vi "Example.vi"() -> ()   [LabVIEW 2016, in "SLSC Switch.lvlib"]
uses:
  SLSC Switch.lvlib
  Classes/slscsl/RelayPosition.ctl
  Classes/SLSC Switch/SLSC Switch.lvclass/SLSC Switch.ctl
  Classes/Relay/Relay.lvclass/Relay.ctl
  Classes/slscsl/RelayAction.ctl
  Classes/Relay/Read relay name.vi
  Classes/SLSC Switch/Initialize (Remote).vi
  Classes/SLSC Switch/Initialize (Local).vi
  Classes/SLSC Switch/Connect Channels (Single).vi
  Classes/SLSC Switch/Connect Channels (Multiple).vi
  Classes/SLSC Switch/Disconnect Channels (Single).vi
  <vilib>/SLSC/Flatten Names (String).vi
  Classes/SLSC Switch/Disconnect Channels (Multiple).vi
  Classes/Switch Action Processor/Switch Action Processor.lvclass
  Classes/SLSC Switch/SLSC Switch.lvclass
  Classes/slscsl/slscsl.lvclass
  <vilib>/SLSC/SLSC.lvlib
panel:
  out "Closed Relays":i32(listbox)
  in  "Remote?":bool
  out "init time":u32
  in  "https?":bool
  in  "Port":u16=8001
  in  "Hostname/IP":string="localhost"
  in  "suffix":string
  in  "Add Topology":bool
  in  "Disconnect All":bool
  out "Active Connections":i32(listbox)
  in  "Tab Control":T1(tab)
  in  "Available Relays":i32[](listbox)
  in  "Open":bool
  in  "Close":bool
  in  "Channel A":i32(listbox)=-1
  in  "Channel B":i32(listbox)=-1
  in  "Disconnect":bool
  in  "Connect":bool
  in  "Add to List":bool
  in  "Connection List":string
  in  "Disconnect Multiple":bool
  in  "Connect Multiple":bool
  in  "Channel B":i32(listbox)=-1
  in  "Channel A":i32(listbox)=-1
  in  "Check MUXList":bool
  in  "Add to MUXList":bool
  in  "Remove from MUXList":bool
  in  "Destinations":i32[](listbox)
  in  "Source":i32(listbox)=-1
  out "Relay Status":cluster{"RelayPosition":T2, "Name":string}[](array[cluster]) {"RelayPosition" items=["Open"=10, "Closed"=11]}
  out "error out":errorcluster
  in  "stop":bool
  in  "error in (no error)":errorcluster
  in  "Topology":string
  in  "device":refnum<k21>
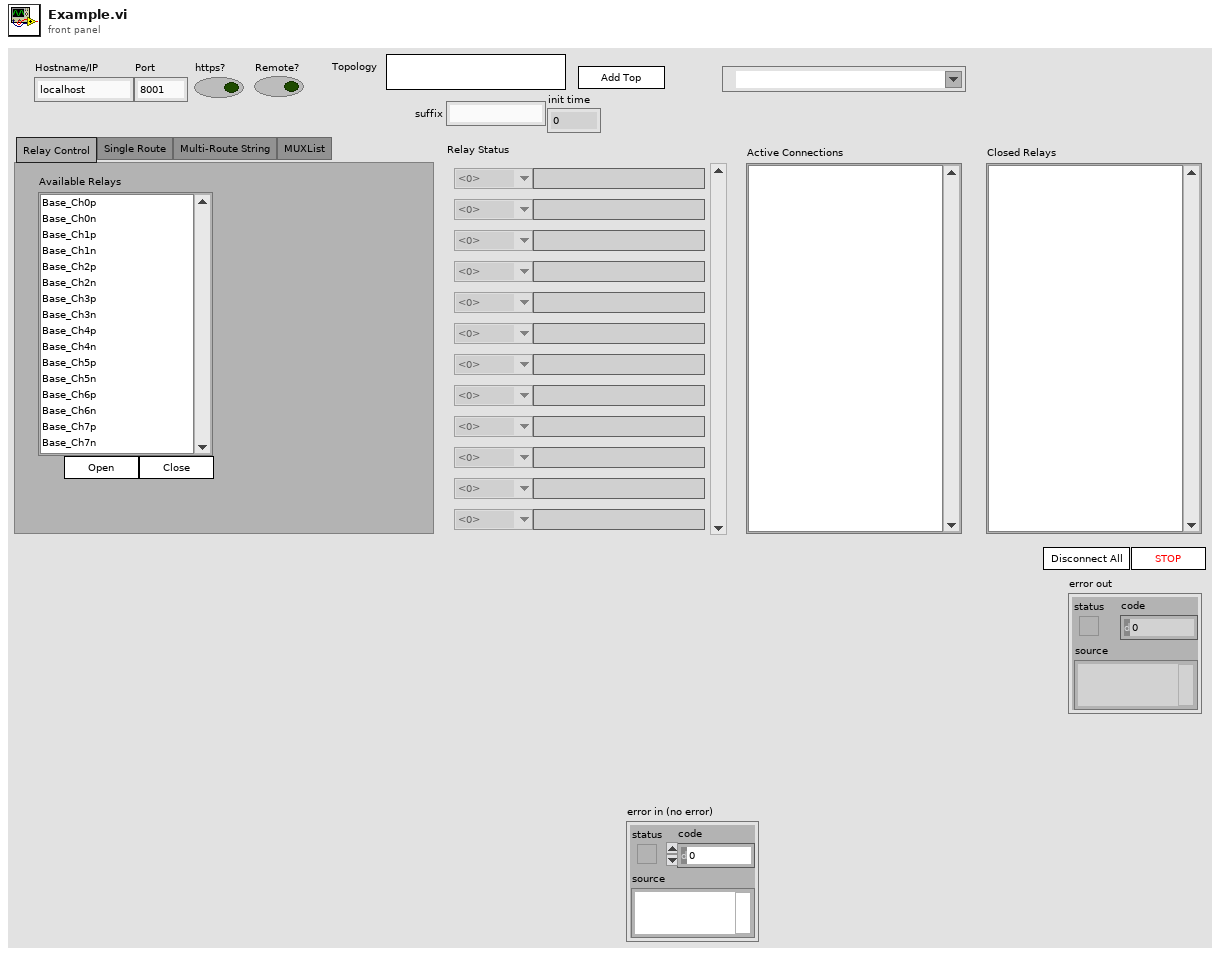
[diagram p1: front panel]
types:
  T1 = enum32{"Relay Control", "Single Route", "Multi-Route String", "MUXList"}
  T2 = typedef "SLSC Switch.lvlib/slscsl.lvclass/RelayPosition.ctl" = i32
  T3 = typedef "SLSC Switch.lvlib/SLSC Switch.lvclass/Connection.ctl" = cluster{"channel 1":string, "channel 2":string}
  T4 = typedef "SLSC Switch.lvlib/slscsl.lvclass/RelayAction.ctl" = u32
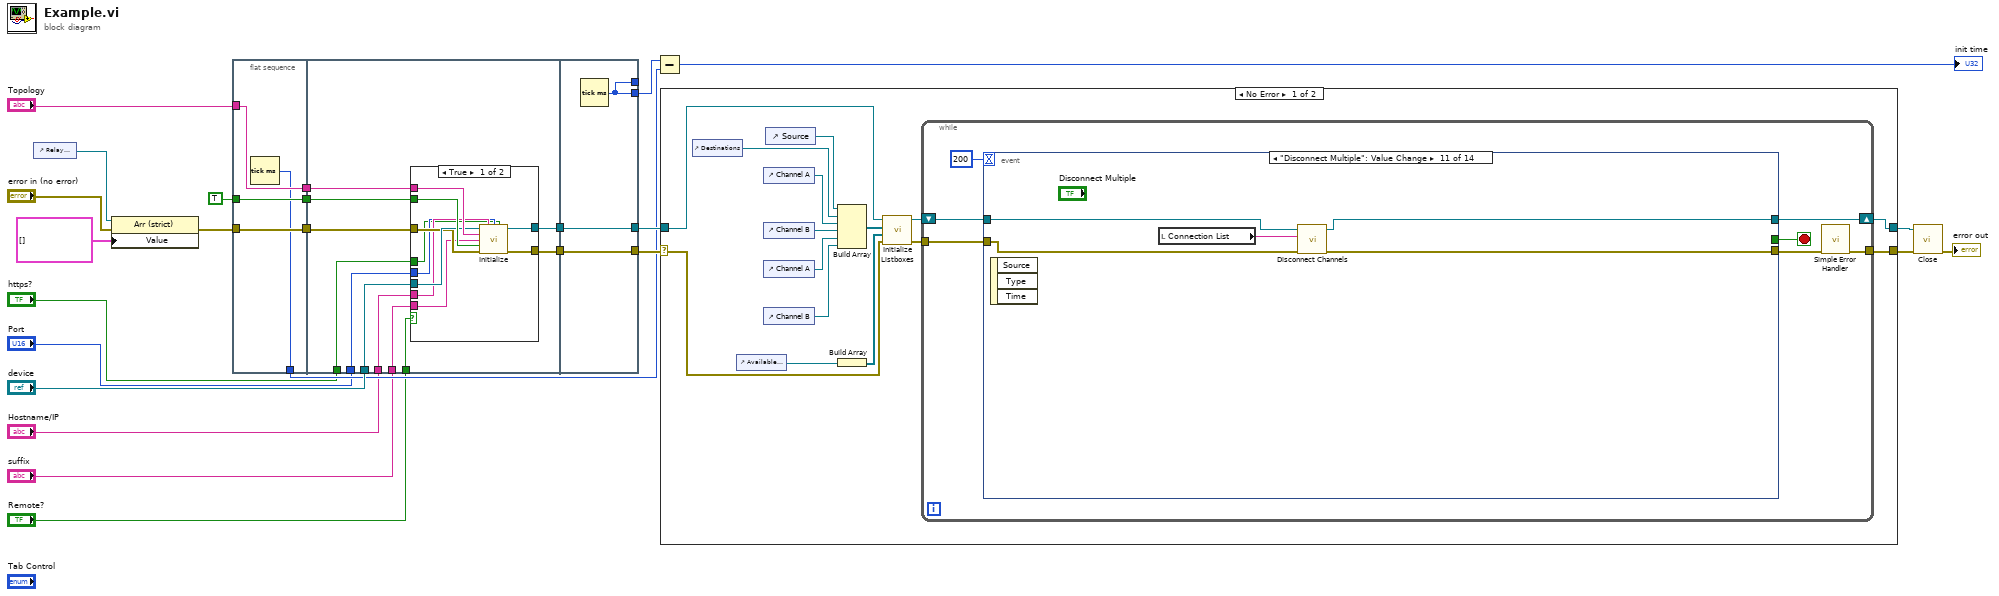
[diagram p0: block diagram]
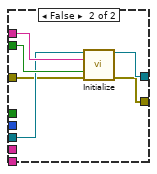
[diagram p2: hidden frame]
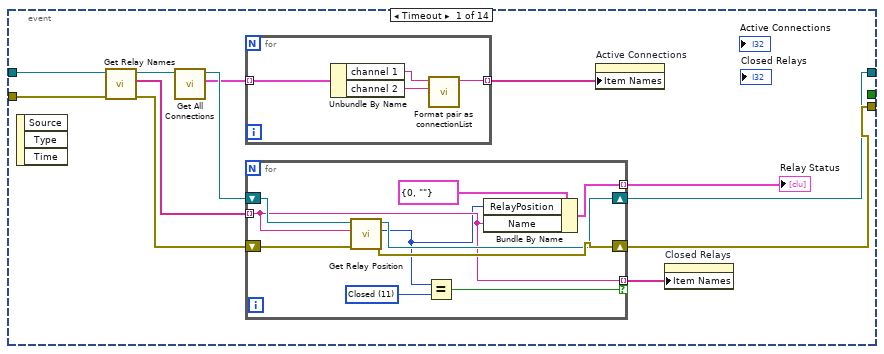
[diagram p3: hidden frame]
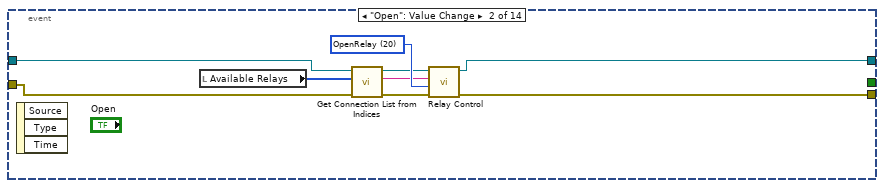
[diagram p4: hidden frame]
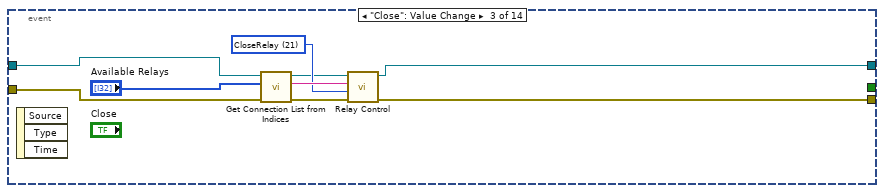
[diagram p5: hidden frame]
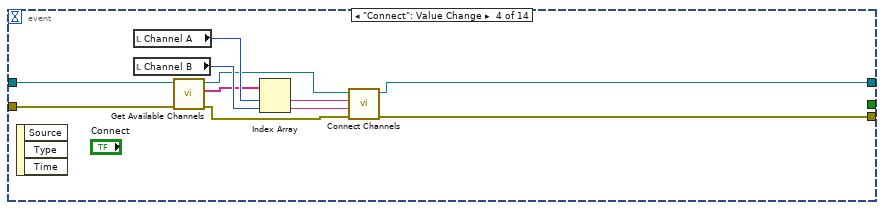
[diagram p6: hidden frame]
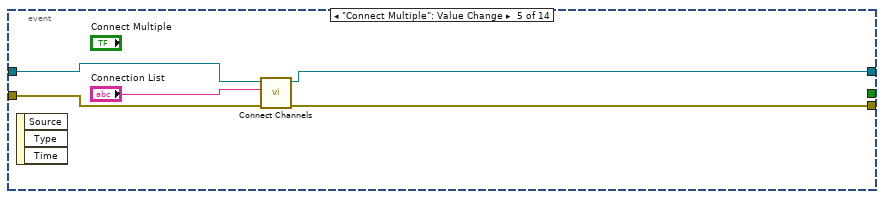
[diagram p7: hidden frame]
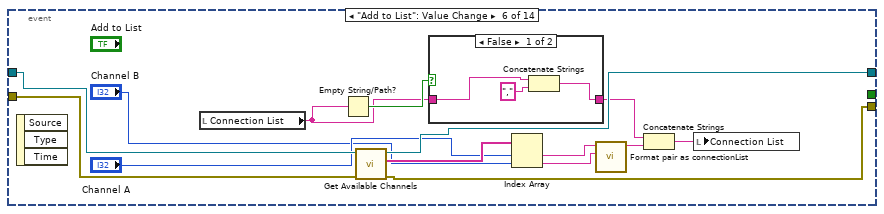
[diagram p8: hidden frame]
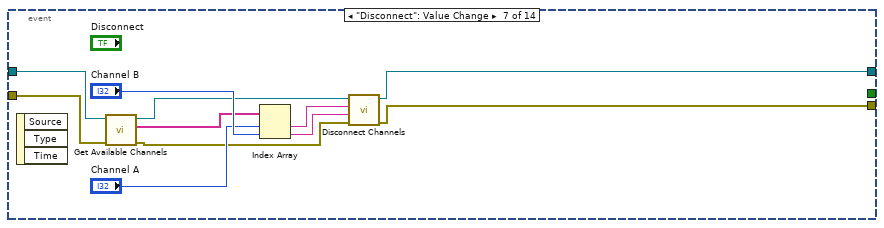
[diagram p10: hidden frame]
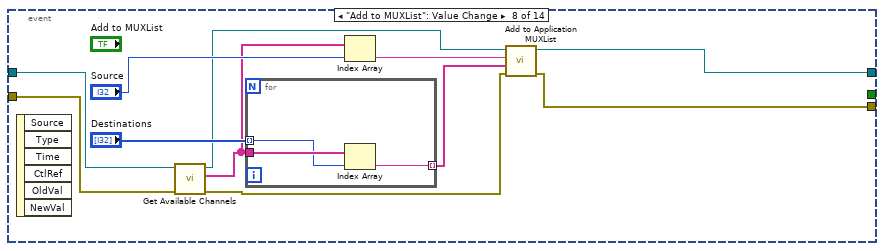
[diagram p11: hidden frame]
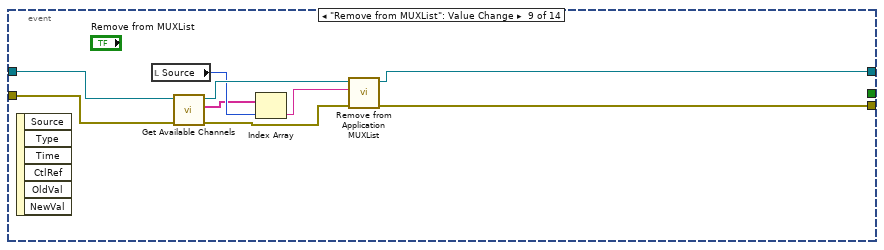
[diagram p12: hidden frame]
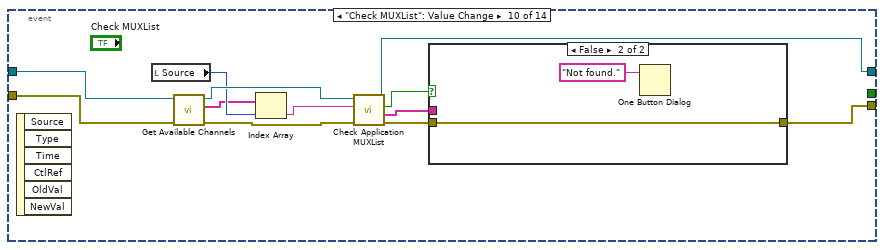
[diagram p13: hidden frame]
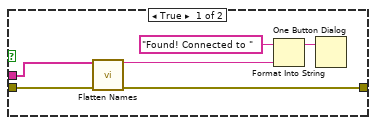
[diagram p14: hidden frame]
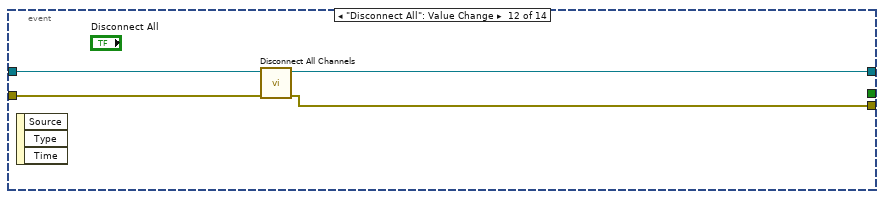
[diagram p15: hidden frame]
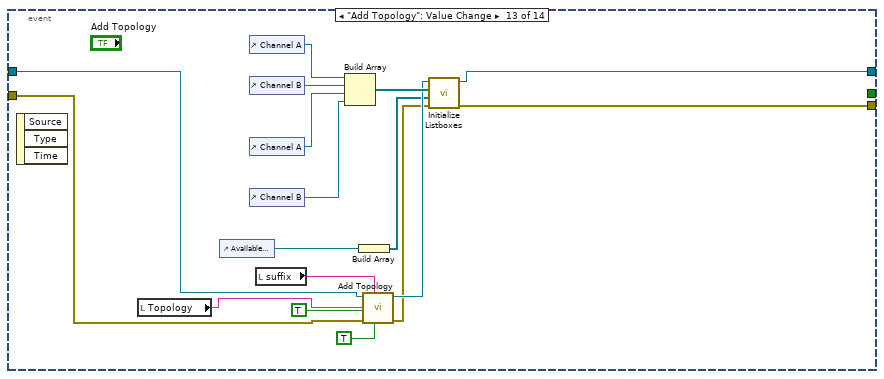
[diagram p16: hidden frame]
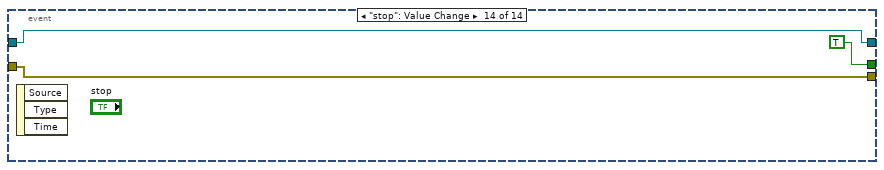
[diagram p17: hidden frame]
diagram:
  n1 = control-ref of="Relay Status"() -> (w18:refnum<vi>)
  n2 = property class="Arr (strict)"(reference=w18, error in="error in (no error)", "Value"=cluster{"RelayPosition":T2, "Name":string}[] []) -> (error out=w16:errorcluster)  [unwired: 1 out]
  n3 = flat-sequence {
    tunnel: w16 -> [w27]
    tunnel: TRUE ("reset device (boolean value)") -> [w28]
    tunnel: "Topology" -> [w29]
    tunnel: [w29] -> w13
    tunnel: [w28] -> w12
    tunnel: [w27] -> w11
    tunnel: [w26] -> w7
    tunnel: "device" -> [w37]
    tunnel: w13 -> [w40]
    tunnel: w12 -> [w38]
    tunnel: w11 -> [w36]
    tunnel: [w39] -> w10
    tunnel: [w35] -> w9
    tunnel: "Remote?" -> [w34]
    tunnel: "Hostname/IP" -> [w33]
    tunnel: "Port" -> [w32]
    tunnel: "https?" -> [w31]
    tunnel: "suffix" -> [w30]
    tunnel: [w58] -> w14
    tunnel: [w59] -> w21
    tunnel: w10 -> [w59]
    tunnel: w9 -> [w58]
    tunnel: [w57] -> _
    tunnel: [w57] -> w8
    frame #0 {
      n4 = Tick Count (ms)() -> (millisecond timer value=w26:u32)
    }
    frame #1 {
      n5 = case shown="True" w34 {
        tunnel: w40 -> [w50 w56]
        tunnel: [w49 w55] -> w39
        tunnel: w38 -> [w48 w54]
        tunnel: w37 -> [w47 w53]
        tunnel: w36 -> [w46 w52]
        tunnel: [w45 w51] -> w35
        tunnel: w33 -> [w44 _]
        tunnel: w32 -> [w43 _]
        tunnel: w31 -> [w42 _]
        tunnel: w30 -> [w41 _]
        frame True {
          n6 = call-poly "Initialize.vi"("device"=w47, "Hostname/IP"=w44, "Port"=w43, "https?"=w42, "Topology"=w50, "topology suffix (none)"=w41, "reset device (boolean value)"=w48, "error in (no error)"=w46) -> ("SLSC Switch out"=w49:refnum<class "SLSC Switch.lvclass">, "error out"=w45:errorcluster)  [unwired: 6 in]
        }
        frame False {
          n7 = call-poly "Initialize.vi"("device"=w53, "Topology"=w56, "reset device (boolean value)"=w54, "error in (no error)"=w52) -> ("SLSC Switch out"=w55:refnum<class "SLSC Switch.lvclass">, "error out"=w51:errorcluster)  [unwired: 10 in]
        }
      }
    }
    frame #2 {
      n8 = Tick Count (ms)() -> (millisecond timer value=w57:u32)
    }
  }
  n9 = Subtract(x=w8, y=w7) -> (x-y=→"init time":u32)
  n10 = case shown="No Error" w14 {
    selector: w14 -> [w64 w243]
    tunnel: [w74 w243] -> w24
    tunnel: [w73 w244] -> w23
    tunnel: w21 -> [w71 w244]
    frame No Error {
      n11 = control-ref of="Destinations"() -> (w60:refnum<vi>)
      n12 = control-ref of="Available Relays"() -> (w65:refnum<vi>)
      n13 = control-ref of="Channel A"() -> (w69:refnum<vi>)
      n14 = control-ref of="Channel B"() -> (w68:refnum<vi>)
      n15 = control-ref of="Channel A"() -> (w67:refnum<vi>)
      n16 = control-ref of="Channel B"() -> (w66:refnum<vi>)
      n17 = control-ref of="Source"() -> (w61:refnum<vi>)
      n18 = Build Array(w61, w60, w69, w68, w67, w66) -> (w63:refnum<vi>[])
      n19 = Build Array(w65) -> (w62:refnum<vi>[])
      n20 = call "Initialize Listboxes.vi"("error in (no error)"=w64, "Relay Boxes"=w62, "Channel Boxes"=w63, "SLSC Switch in"=w71) -> ("error out"=w70:errorcluster, "SLSC Switch out"=w72:refnum<class "SLSC Switch.lvclass">)  [unwired: 6 in]
      n21 = while {
        shift-right: [w79] -> w73
        shift-left: w72 -> [w80]
        tunnel: w70 -> [w81]
        tunnel: [w75] -> w74
        stop <- w77 stop-if-true
        n22 = event shown="[10] \"Disconnect Multiple\": Value Change" {
          selector: _ -> [_ _ _ _ _ _ _ _ _ _ _ _ _ _]
          dyn-events: _ -> [_ _ _ _ _ _ _ _ _ _ _ _ _ _]
          timeout: 200 -> [_ _ _ _ _ _ _ _ _ _ _ _ _ _]
          tunnel: w81 -> [w84 w109 w118 w127 w138 w154 w161 w172 w186 w199 w216 w222 w238 w242]
          tunnel: [w93 w116 w125 w135 w137 w152 w169 w173 w189 w194 w215 w219 w226 w242] -> w76
          tunnel: w80 -> [w87 w113 w120 w130 w141 w155 w164 w181 w193 w205 w218 w221 w239 w241]
          tunnel: [w92 w115 w124 w136 w140 w153 w170 w176 w191 w203 w217 w220 w228 w241] -> w79
          tunnel: [_ _ _ _ _ _ _ _ _ _ _ _ _ TRUE] -> w77
          event Timeout {
            n23 = event-data() -> ()  [unwired: 1 in, 3 out]
            n24 = call "Get Relay Names.vi"("error in (no error)"=w84, "SLSC Switch in"=w87) -> ("error out"=w83:errorcluster, "Relay Names"=w85:string[], "SLSC Switch out"=w86:refnum<class "SLSC Switch.lvclass">)  [unwired: 7 in]
            n25 = call "Get All Connections.vi"("Route Manager in"=w86) -> ("connections"=w89:T3[], "Route Manager out"=w91:refnum<class "SLSC Switch.lvclass">)  [unwired: 9 in]
            n26 = for {
              tunnel: w89 -> [w97] mode=indexing
              tunnel: [w94] -> w88 mode=indexing
              n27 = Unbundle By Name(w97) -> ("channel 1"=w96:string, "channel 2"=w95:string)
              n28 = call "Format pair as connectionList.vi"("channel in"=w95, "channel 1"=w96) -> ("connectionList"=w94:string)  [unwired: 9 in]
            }
            n29 = for {
              shift-right: [w104] -> w92
              shift-left: w91 -> [w107]
              shift-right: [w105] -> w93
              shift-left: w83 -> [w106]
              tunnel: [w102] -> w90 mode=indexing
              tunnel: w85 -> [w101] mode=indexing
              tunnel: [w101] -> w82 mode=indexing if=w98
              w99 = T2 11 items=["Open"=10, "Closed"=11] ("y")
              n30 = call "Get Relay Position.vi"("error in (no error)"=w106, "relay name"=w101, "SLSC Switch in"=w107) -> ("error out"=w105:errorcluster, "position"=w100:T2, "SLSC Switch out"=w104:refnum<class "SLSC Switch.lvclass">)  [unwired: 6 in]
              n31 = Equal?(x=w100, y=w99) -> (x = y?=w98:bool)
              n32 = Bundle By Name(cluster=cluster{"RelayPosition":T2, "Name":string} {"RelayPosition"=0, "Name"=""} ("Relay"), "RelayPosition"=w100, "Name"=w101) -> (w102:cluster{"RelayPosition":T2, "Name":string})
            }
            "Relay Status" <- w90
            n33 = property on="Active Connections" class="LstBox (strict)"("Item Names"=w88) -> ()  [unwired: 2 in, 2 out]
            n34 = property on="Closed Relays" class="LstBox (strict)"("Item Names"=w82) -> ()  [unwired: 2 in, 2 out]
          }
          event "Open": Value Change {
            w114 = T4 20 items=["CloseRelay"=21, "OpenRelay"=20] ("RelayAction")
            n35 = event-data() -> ()  [unwired: 1 in, 3 out]
            n36 = local read "Available Relays"() -> (w110:i32[])
            n37 = call "Get Connection List from Indices.vi"("error in (no error)"=w109, "Available Relays"=w110, "SLSC Switch in"=w113) -> ("error out"=w108:errorcluster, "String"=w111:string, "SLSC Switch out"=w112:refnum<class "SLSC Switch.lvclass">)  [unwired: 6 in]
            n38 = call "Relay Control.vi"("error in (no error)"=w108, "relay action"=w114, "relay names"=w111, "SLSC Switch in"=w112) -> ("error out"=w116:errorcluster, "SLSC Switch out"=w115:refnum<class "SLSC Switch.lvclass">)  [unwired: 6 in]
          }
          event "Close": Value Change {
            w122 = T4 21 items=["CloseRelay"=21, "OpenRelay"=20] ("RelayAction")
            n39 = event-data() -> ()  [unwired: 1 in, 3 out]
            n40 = call "Get Connection List from Indices.vi"("error in (no error)"=w118, "Available Relays"="Available Relays", "SLSC Switch in"=w120) -> ("error out"=w117:errorcluster, "String"=w123:string, "SLSC Switch out"=w119:refnum<class "SLSC Switch.lvclass">)  [unwired: 6 in]
            n41 = call "Relay Control.vi"("error in (no error)"=w117, "relay action"=w122, "relay names"=w123, "SLSC Switch in"=w119) -> ("error out"=w125:errorcluster, "SLSC Switch out"=w124:refnum<class "SLSC Switch.lvclass">)  [unwired: 6 in]
          }
          event "Connect": Value Change {
            n42 = event-data() -> ()  [unwired: 1 in, 3 out]
            n43 = local read "Channel A"() -> (w132:i32)
            n44 = local read "Channel B"() -> (w131:i32)
            n45 = call "Get Available Channels.vi"("error in (no error)"=w127, "SLSC Switch in"=w130) -> ("error out"=w126:errorcluster, "Channels"=w128:string[], "SLSC Switch out"=w129:refnum<class "SLSC Switch.lvclass">)  [unwired: 7 in]
            n46 = Index Array(array=w128, index #1=w132, index #2=w131) -> (element #1=w134:string, element #2=w133:string)
            n47 = call-poly "Connect Channels.vi"("error in (no error)"=w126, "channel 2"=w133, "channel 1"=w134, "SLSC Switch in"=w129) -> ("error out"=w135:errorcluster, "SLSC Switch out"=w136:refnum<class "SLSC Switch.lvclass">)  [unwired: 6 in]
          }
          event "Connect Multiple": Value Change {
            n48 = event-data() -> ()  [unwired: 1 in, 3 out]
            n49 = call-poly "Connect Channels.vi"("error in (no error)"=w138, "connection list"="Connection List", "SLSC Switch in"=w141) -> ("error out"=w137:errorcluster, "SLSC Switch out"=w140:refnum<class "SLSC Switch.lvclass">)  [unwired: 7 in]
          }
          event "Add to List": Value Change {
            n50 = event-data() -> ()  [unwired: 1 in, 3 out]
            n51 = local read "Connection List"() -> (w149:string)
            n52 = Empty String/Path?(string/path=w149) -> (empty?=w150:bool)
            n53 = call "Get Available Channels.vi"("error in (no error)"=w154, "SLSC Switch in"=w155) -> ("error out"=w152:errorcluster, "Channels"=w151:string[], "SLSC Switch out"=w153:refnum<class "SLSC Switch.lvclass">)  [unwired: 7 in]
            n54 = case shown="False" w150 {
              tunnel: w149 -> [w158 w159]
              tunnel: [w156 w159] -> w148
              frame False {
                n55 = Concatenate Strings(w158, "," ("string")) -> (w156:string)
              }
              frame True {
              }
            }
            n56 = Index Array(array=w151, index #1="Channel A", index #2="Channel B") -> (element #1=w147:string, element #2=w146:string)
            n57 = call "Format pair as connectionList.vi"("channel in"=w146, "channel 1"=w147) -> ("connectionList"=w145:string)  [unwired: 9 in]
            n58 = Concatenate Strings(w148, w145) -> (w144:string)
            n59 = local write "Connection List"(w144) -> ()
          }
          event "Disconnect": Value Change {
            n60 = event-data() -> ()  [unwired: 1 in, 3 out]
            n61 = call "Get Available Channels.vi"("error in (no error)"=w161, "SLSC Switch in"=w164) -> ("error out"=w160:errorcluster, "Channels"=w163:string[], "SLSC Switch out"=w162:refnum<class "SLSC Switch.lvclass">)  [unwired: 7 in]
            n62 = Index Array(array=w163, index #1="Channel A", index #2="Channel B") -> (element #1=w168:string, element #2=w167:string)
            n63 = call-poly "Disconnect Channels.vi"("error in (no error)"=w160, "channel 2"=w167, "channel 1"=w168, "SLSC Switch in"=w162) -> ("error out"=w169:errorcluster, "SLSC Switch out"=w170:refnum<class "SLSC Switch.lvclass">)  [unwired: 6 in]
          }
          event "Add to MUXList": Value Change {
            n64 = event-data() -> ()  [unwired: 1 in, 6 out]
            n65 = call "Get Available Channels.vi"("error in (no error)"=w172, "SLSC Switch in"=w181) -> ("error out"=w171:errorcluster, "Channels"=w178:string[], "SLSC Switch out"=w177:refnum<class "SLSC Switch.lvclass">)  [unwired: 7 in]
            n66 = for {
              tunnel: "Destinations" -> [w182] mode=indexing
              tunnel: w178 -> [w184]
              tunnel: [w183] -> w174 mode=indexing
              n67 = Index Array(array=w184, index=w182) -> (element=w183:string)
            }
            n68 = Index Array(array=w178, index="Source") -> (element=w175:string)
            n69 = call "Add to Application MUXList.vi"("error in (no error)"=w171, "Destinations"=w174, "Source"=w175, "SLSC Switch in"=w177) -> ("error out"=w173:errorcluster, "SLSC Switch out"=w176:refnum<class "SLSC Switch.lvclass">)  [unwired: 5 in, 1 out]
          }
          event "Remove from MUXList": Value Change {
            n70 = event-data() -> ()  [unwired: 1 in, 6 out]
            n71 = local read "Source"() -> (w188:i32)
            n72 = call "Get Available Channels.vi"("error in (no error)"=w186, "SLSC Switch in"=w193) -> ("error out"=w185:errorcluster, "Channels"=w187:string[], "SLSC Switch out"=w192:refnum<class "SLSC Switch.lvclass">)  [unwired: 7 in]
            n73 = Index Array(array=w187, index=w188) -> (element=w190:string)
            n74 = call "Remove from Application MUXList.vi"("error in (no error)"=w185, "Source"=w190, "SLSC Switch in"=w192) -> ("error out"=w189:errorcluster, "SLSC Switch out"=w191:refnum<class "SLSC Switch.lvclass">)  [unwired: 7 in]
          }
          event "Check MUXList": Value Change {
            n75 = event-data() -> ()  [unwired: 1 in, 6 out]
            n76 = local read "Source"() -> (w201:i32)
            n77 = call "Get Available Channels.vi"("error in (no error)"=w199, "SLSC Switch in"=w205) -> ("error out"=w198:errorcluster, "Channels"=w200:string[], "SLSC Switch out"=w204:refnum<class "SLSC Switch.lvclass">)  [unwired: 7 in]
            n78 = Index Array(array=w200, index=w201) -> (element=w202:string)
            n79 = call "Check Application MUXList.vi"("error in (no error)"=w198, "Source"=w202, "SLSC Switch in"=w204) -> ("error out"=w195:errorcluster, "Destinations"=w197:string[], "found?"=w196:bool, "SLSC Switch out"=w203:refnum<class "SLSC Switch.lvclass">)  [unwired: 4 in, 1 out]
            n80 = case shown="False" w196 {
              tunnel: w197 -> [w209 _]
              tunnel: w195 -> [w207 w212]
              tunnel: [w206 w212] -> w194
              frame True {
                n81 = call-poly <vilib>:"Flatten Names.vi"("names in"=w209, "error in (no error)"=w207) -> ("names out"=w208:string, "error out"=w206:errorcluster)  [unwired: 12 in]
                n82 = Format Into String(initial string="Found! Connected to ", w208) -> (resulting string=w210:string)  [unwired: 2 in, 1 out]
                n83 = One Button Dialog(message=w210) -> ()  [unwired: 1 in, 1 out]
              }
              frame False {
                n84 = One Button Dialog(message="Not found.") -> ()  [unwired: 1 in, 1 out]
              }
            }
          }
          event "Disconnect Multiple": Value Change {
            n85 = event-data() -> ()  [unwired: 1 in, 3 out]
            n86 = local read "Connection List"() -> (w214:string)
            n87 = call-poly "Disconnect Channels.vi"("error in (no error)"=w216, "disconnection list"=w214, "SLSC Switch in"=w218) -> ("error out"=w215:errorcluster, "SLSC Switch out"=w217:refnum<class "SLSC Switch.lvclass">)  [unwired: 7 in]
          }
          event "Disconnect All": Value Change {
            n88 = event-data() -> ()  [unwired: 1 in, 3 out]
            n89 = call "Disconnect All Channels.vi"("error in (no error)"=w222, "SLSC Switch in"=w221) -> ("error out"=w219:errorcluster, "SLSC Switch out"=w220:refnum<class "SLSC Switch.lvclass">)  [unwired: 8 in]
          }
          event "Add Topology": Value Change {
            n90 = event-data() -> ()  [unwired: 1 in, 3 out]
            n91 = local read "Topology"() -> (w236:string)
            n92 = control-ref of="Available Relays"() -> (w234:refnum<vi>)
            n93 = control-ref of="Channel A"() -> (w230:refnum<vi>)
            n94 = control-ref of="Channel B"() -> (w231:refnum<vi>)
            n95 = control-ref of="Channel A"() -> (w232:refnum<vi>)
            n96 = control-ref of="Channel B"() -> (w233:refnum<vi>)
            n97 = local read "suffix"() -> (w223:string)
            n98 = Build Array(w230, w231, w232, w233) -> (w235:refnum<vi>[])
            n99 = Build Array(w234) -> (w225:refnum<vi>[])
            n100 = call "Add Topology.vi"("Append to Active?"=TRUE, "topology suffix (none)"=w223, "error in (no error)"=w238, "reset device (boolean value)"=TRUE, "Topology"=w236, "SLSC Switch in"=w239) -> ("error out"=w227:errorcluster, "SLSC Switch out"=w229:refnum<class "SLSC Switch.lvclass">)  [unwired: 4 in]
            n101 = call "Initialize Listboxes.vi"("error in (no error)"=w227, "Relay Boxes"=w225, "Channel Boxes"=w235, "SLSC Switch in"=w229) -> ("error out"=w226:errorcluster, "SLSC Switch out"=w228:refnum<class "SLSC Switch.lvclass">)  [unwired: 6 in]
          }
          event "stop": Value Change {
            n102 = event-data() -> ()  [unwired: 1 in, 3 out]
          }
        }
        n103 = call <vilib>:"Simple Error Handler.vi"("error in (no error)"=w76) -> ("error out"=w75:errorcluster)  [unwired: 4 in, 4 out]
      }
    }
    frame Error {
    }
  }
  n104 = call "Close.vi"("error in (no error)"=w24, "SLSC Switch in"=w23) -> ("error out"=→"error out":errorcluster)  [unwired: 9 in]
